vi "ResizeCluster.vi"(11 "Cluster in":refnum<vi>) -> ()   [LabVIEW 2023]
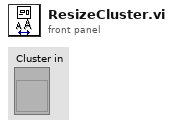
[diagram p1: front panel]
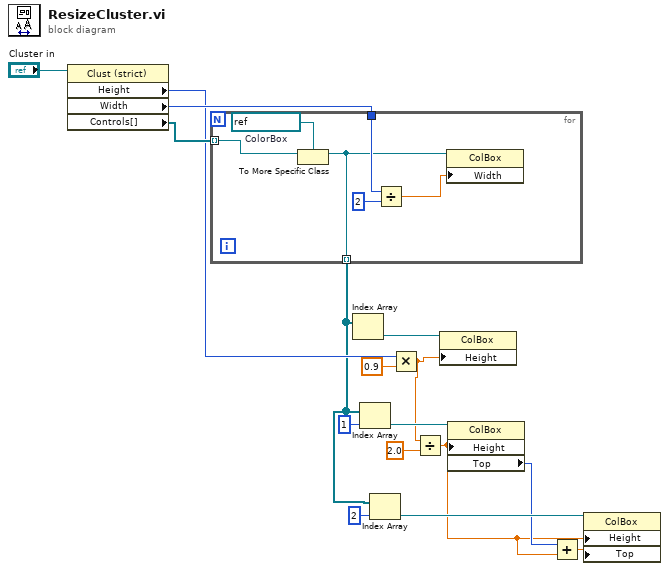
[diagram p0: block diagram]
diagram:
  n1 = property class="Clust (strict)"(reference="Cluster in") -> ("Height"=w12:u32, "Width"=w15:u32, "Controls[]"=w14:refnum<vi>[])  [unwired: 1 in, 2 out]
  n2 = for {
    tunnel: w15 -> [w21]
    tunnel: w14 -> [w18] mode=indexing
    tunnel: [w17] -> w4 mode=indexing
    w22 = refnum<vi> refnum  # ColorBox
    n3 = To More Specific Class(target class=w22, reference=w18) -> (specific class reference=w17:refnum<vi>)  [unwired: 1 in, 1 out]
    n4 = Divide(x=w21, y=u32 2) -> (x/y=w20:dbl)
    n5 = property class="ColBox"(reference=w17, "Width"=w20) -> ()  [unwired: 1 in, 2 out]
  }
  n6 = Index Array(array=w4) -> (element=w13:refnum<vi>)  [unwired: 1 in]
  n7 = Index Array(array=w4, index=1) -> (element=w9:refnum<vi>)
  n8 = Index Array(array=w4, index=2) -> (element=w6:refnum<vi>)
  n9 = Multiply(x=w12, y=0.9) -> (x*y=w8:dbl)
  n10 = Divide(x=w8, y=2.0) -> (x/y=w1:dbl)
  n11 = property class="ColBox"(reference=w13, "Height"=w8) -> ()  [unwired: 1 in, 2 out]
  n12 = property class="ColBox"(reference=w9, "Height"=w1) -> ("Top"=w2:i32)  [unwired: 1 in, 2 out]
  n13 = Add(x=w2, y=w1) -> (x+y=w3:dbl)
  n14 = property class="ColBox"(reference=w6, "Height"=w1, "Top"=w3) -> ()  [unwired: 1 in, 2 out]
